vi "CreateSimulatedData.vi"(8 "error in (no error)":errorcluster, 10 "index":i32) -> (0 "error out":errorcluster, 2 "channel status":string, 3 "value":dbl)   [LabVIEW 2017, in "ScanEngine.lvlib"]
uses:
  <vilib>/addons/InsightCM/Devices/Shared/Common/ScanEngine/ScanEngine.lvlib
  <vilib>/addons/InsightCM/Devices/Shared/Common/ScanEngine/subVIs/SimulatedConfigRefGlobal.vi
  <vilib>/addons/InsightCM/Utilities/ChannelStatus/ChannelStatus.lvlib
panel:
  in  "TestChStatus":bool
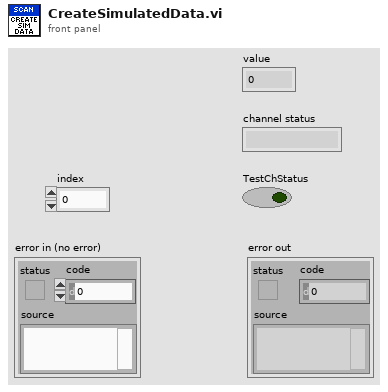
[diagram p1: front panel]
types:
  T1 = typedef "ScanEngine.lvlib/SimConfigRefs.ctl" = cluster{"Scan Engine Config":refnum<vi>}
  T2 = typedef "SimulatedData.ctl" = cluster{"Channel":string, "Value":dbl, "Random":bool, "Delta":dbl}
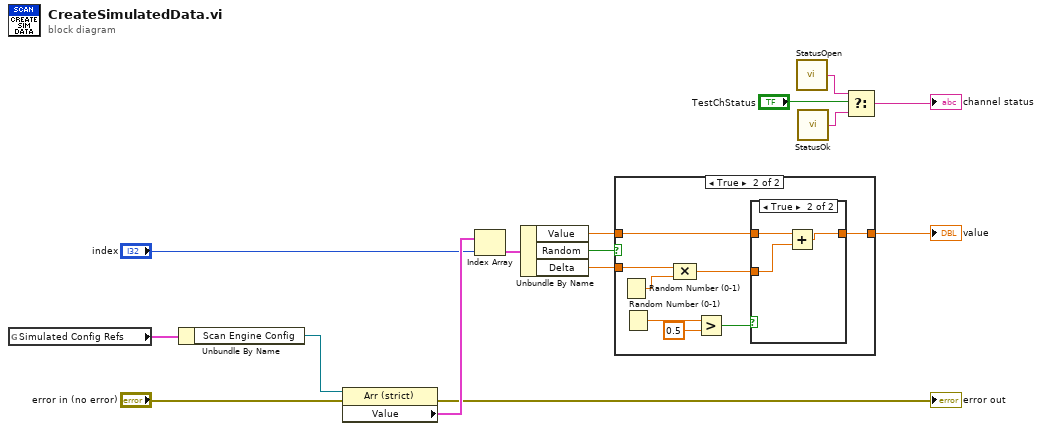
[diagram p0: block diagram]
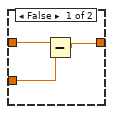
[diagram p3: hidden frame]
diagram:
  n1 = global read "SimulatedConfigRefGlobal.vi" "Simulated Config Refs"() -> (w1:T1)
  n2 = Unbundle By Name(w1) -> ("Scan Engine Config"=w10:refnum<vi>)
  n3 = property class="Arr (strict)"(reference=w10, error in="error in (no error)") -> (error out=→"error out":errorcluster, "Value"=w9:T2[])  [unwired: 1 out]
  n4 = Index Array(array=w9, index="index") -> (element=w15:T2)
  n5 = Unbundle By Name(w15) -> ("Value"=w13:dbl, "Random"=w12:bool, "Delta"=w11:dbl)
  n6 = case shown="True" w12 {
    tunnel: w11 -> [_ w24]
    tunnel: w13 -> [w16 w22]
    tunnel: [w16 w17] -> w14
    frame False {
    }
    frame True {
      n7 = Random Number (0-1)() -> (number: 0 to 1=w23:dbl)
      n8 = Random Number (0-1)() -> (number: 0 to 1=w21:dbl)
      n9 = Compound Arithmetic op=MULTIPLY(w24, w23) -> (w18:dbl)
      n10 = Greater?(x=w21, y=0.5) -> (0:w19:bool)
      n11 = case shown="True" w19 {
        tunnel: w22 -> [w27 w30]
        tunnel: w18 -> [w26 w29]
        tunnel: [w25 w28] -> w17
        frame False {
          n12 = Subtract(x=w27, y=w26) -> (x-y=w25:dbl)
        }
        frame True {
          n13 = Add(x=w30, y=w29) -> (x+y=w28:dbl)
        }
      }
    }
  }
  "value" <- w14
  n14 = call <vilib>:"StatusOpen.vi"() -> ("status"=w3:string)  [unwired: 5 in]
  n15 = call <vilib>:"StatusOk.vi"() -> ("status"=w4:string)  [unwired: 5 in]
  n16 = Select(t=w3, s="TestChStatus", f=w4) -> (s? t:f=→"channel status":string)
